vi "出队.vi"(10 "数组输入":cluster{"x":dbl, "y":dbl}[](array[cluster]), 11 "地图":u32[][](array[colorbox])) -> (2 "数组输出":cluster{"x":dbl, "y":dbl}[](array[cluster]), 3 "地图 2":u32[][](array[colorbox]))   [LabVIEW 2012]
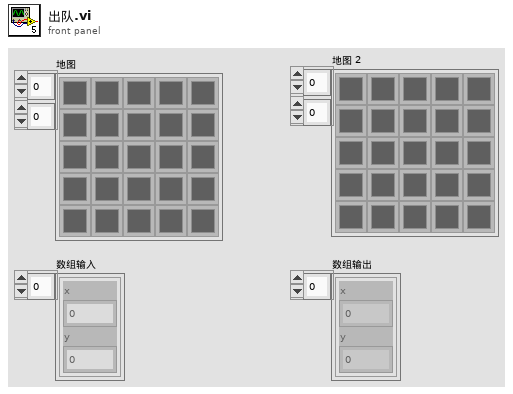
[diagram p1: front panel]
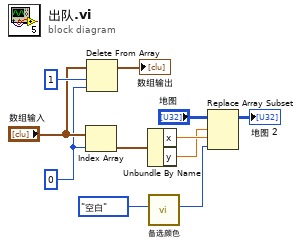
[diagram p0: block diagram]
diagram:
  w2 = 0 ("索引")
  n1 = Index Array(array="数组输入", index=w2) -> (element=w1:cluster{"x":dbl, "y":dbl})
  n2 = Delete From Array(array="数组输入", length=1 ("长度"), index=w2) -> (array with subset deleted=→"数组输出":cluster{"x":dbl, "y":dbl}[])  [unwired: 1 out]
  n3 = Unbundle By Name(w1) -> ("x"=w10:dbl, "y"=w9:dbl)
  n4 = call "备选颜色.vi"("索引2"=enum16{"空白", "蛇", "食物", "墙", "传送门"}."空白") -> ("颜色2"=w7:u32)  [unwired: 9 in, 1 out]
  n5 = Replace Array Subset(array="地图", new element=w7, index (row)=w9, index (col)=w10) -> (→"地图 2":u32[][])
